vi "CounterCountEdgePulseSync.vi"() -> ()   [LabVIEW 2023]
uses:
  <vilib>/Utility/error.llb/DialogType.ctl
  <vilib>/DAQmx/read.llb/DAQmx Read (Counter 1D DBL 1Chan NSamp).vi
  <vilib>/DAQmx/create/channels.llb/DAQmx Create Channel (CI-Count Edges).vi
  <vilib>/DAQmx/create/channels.llb/DAQmx Create Channel (CO-Pulse Generation-Time).vi
  <vilib>/DAQmx/create/channels.llb/DAQmx Create Channel (AI-Voltage-Basic).vi
  <vilib>/DAQmx/configure/timing.llb/DAQmx Timing (Sample Clock).vi
  <vilib>/DAQmx/configure/timing.llb/DAQmx Timing (Implicit).vi
  <vilib>/DAQmx/miscellaneous.llb/DAQmx Fill In Error Info.vi
  <resource>/objmgr/daqmx.rc
panel:
  in  "# of pulses":i32=1000
  in  "Pulse Output terminal":tag
  in  "CI.CountEdges.Term":tag
  out "data":dbl[](array[numeric]) caption="Counter 0 Data" format="%0.2f"
  in  "Sample Clock Source":tag="/Dev1/ai/SampleClock"
  in  "rate":dbl=1000.0 format="%0.2f"
  in  "Physical Channel":tag="Dev1/ai0"
  in  "active edge":i32(ring)=10280 items=["Rising"=10280, "Falling"=10171]
  in  "Physical Channel":tag="Dev1/ctr1"
  in  "Physical Channel":tag="Dev1/ctr0"
  in  "stop":bool
  # "Analog Channel Properties"
  # "Counter 0 Channel Properties"
  # "Counter 1 Channel Properties"
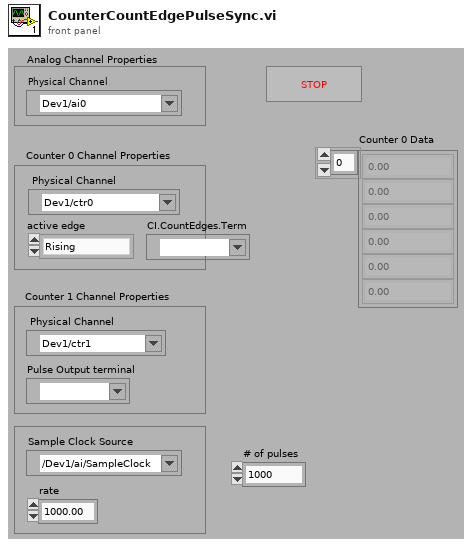
[diagram p1: front panel]
types:
  T1 = typedef "DialogType.ctl" = u16
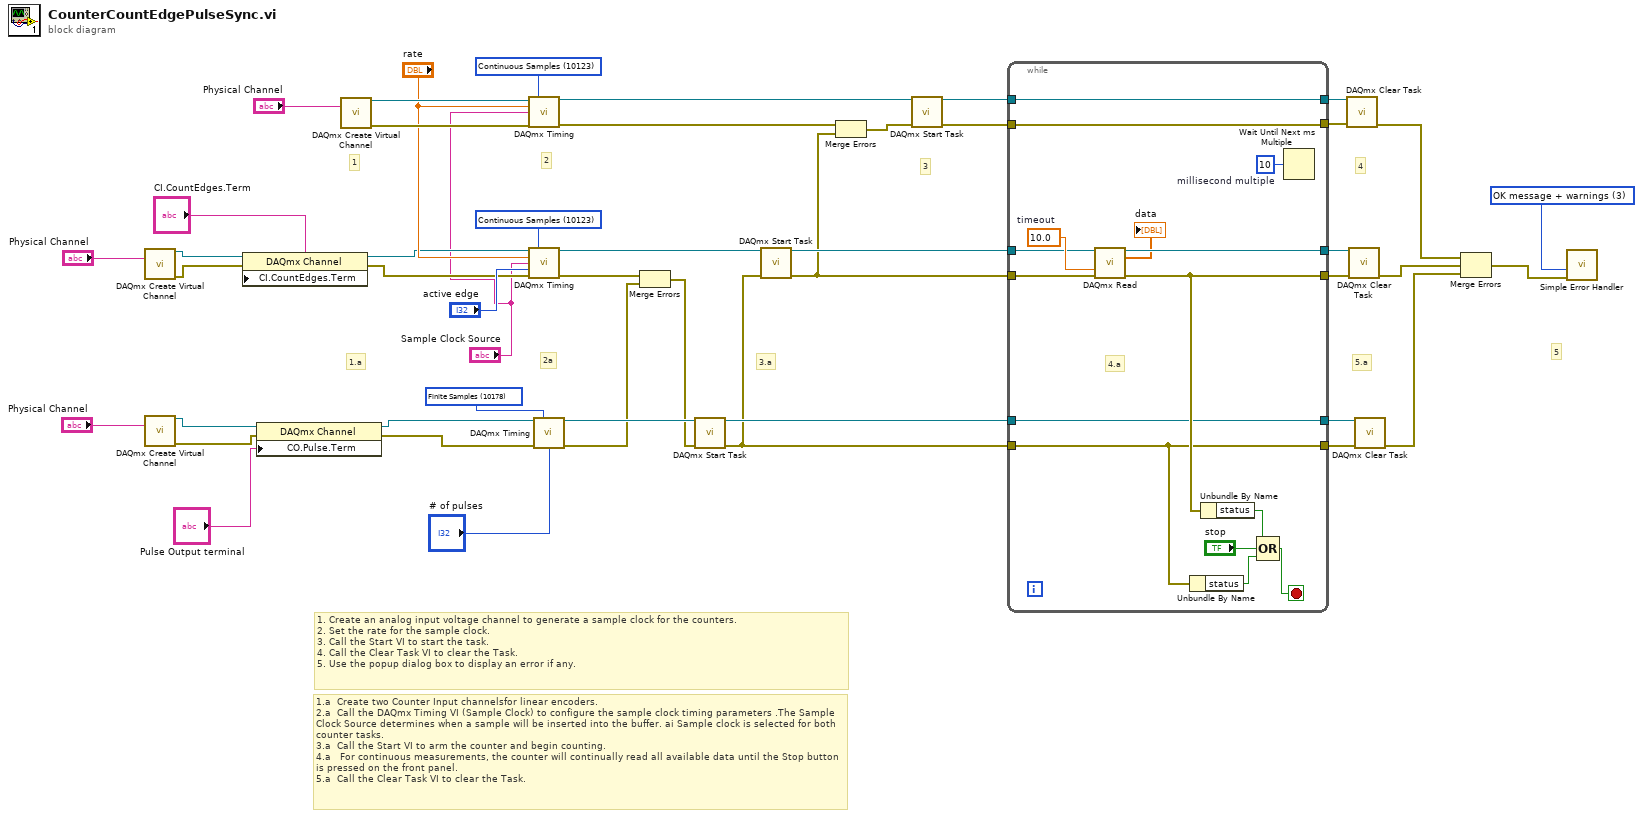
[diagram p0: block diagram]
diagram:
  w13 = 10123 items=["Finite Samples"=10178, "Continuous Samples"=10123, "Hardware Timed Single Point"=12522] ("sample mode")
  w14 = 10178 items=["Finite Samples"=10178, "Continuous Samples"=10123, "Hardware Timed Single Point"=12522] ("sample mode")
  w15 = 10123 items=["Finite Samples"=10178, "Continuous Samples"=10123, "Hardware Timed Single Point"=12522] ("sample mode")
  w33 = T1 3 items=["no dialog", "OK message", "continue or stop message", "OK message + warnings", "continue/stop + warnings"] ("type of dialog (OK msg:1)")
  # "1. Create an analog input voltage channel to generate a sample clock for the counters.\n2. Set the rate for the sample clock.\n3. Call the Start VI to start the task.\n4. Call the Clear Task VI to clear the Task.\n5. Use the popup dialog box to display an error if any."
  # "5"
  # "1.a  Create two Counter Input channelsfor linear encoders. \n2.a  Call the DAQmx Timing VI (Sample Clock) to configure the sample clock timing parameters .The Sample Clock Source determines when a sample will be inserted into the buffer. ai Sample clock is selected for both counter tasks.\n3.a  Call the Start VI to arm the counter and begin counting.\n4.a   For continuous measurements, the counter will continually read all available data until the Stop button is pressed on the front panel.\n5.a  Call the Clear Task VI to clear the Task."
  # "5.a"
  # "3.a"
  # "2a"
  # "1.a"
  # "4"
  # "3"
  # "2"
  # "1"
  n1 = call-poly <vilib>:"DAQmx Create Virtual Channel.vi"("counter"="Physical Channel") -> ("task out"=w12:refnum<k21>, "error out"=w9:errorcluster)  [unwired: 6 in, 7 out]
  n2 = call-poly <vilib>:"DAQmx Create Virtual Channel.vi"("counter"="Physical Channel") -> ("task out"=w7:refnum<k21>, "error out"=w4:errorcluster)  [unwired: 8 in, 5 out]
  n3 = property class="DAQmx Channel"(reference=w12, error in=w9, "CI.CountEdges.Term"="CI.CountEdges.Term") -> (reference out=w11:refnum<k21>, error out=w10:errorcluster)
  n4 = property class="DAQmx Channel"(reference=w7, error in=w4, "CO.Pulse.Term"="Pulse Output terminal") -> (reference out=w6:refnum<k21>, error out=w5:errorcluster)
  n5 = call-poly <vilib>:"DAQmx Create Virtual Channel.vi"("physical channels"="Physical Channel") -> ("task out"=w47:refnum<k21>, "error out"=w46:errorcluster)  [unwired: 8 in, 5 out]
  n6 = call-poly <vilib>:"DAQmx Timing.vi"("task/channels in"=w47, "sample mode"=w15, "rate"="rate", "source"="Sample Clock Source", "error in"=w46) -> ("task out"=w41:refnum<k21>, "error out"=w37:errorcluster)  [unwired: 2 in, 7 out]
  n7 = call-poly <vilib>:"DAQmx Timing.vi"("task/channels in"=w11, "sample mode"=w13, "rate"="rate", "source"="Sample Clock Source", "active edge"="active edge", "error in"=w10) -> ("task out"=w43:refnum<k21>, "error out"=w40:errorcluster)  [unwired: 1 in, 7 out]
  n8 = call-poly <vilib>:"DAQmx Timing.vi"("task/channels in"=w6, "sample mode"=w14, "samples per channel"="# of pulses", "error in"=w5) -> ("task out"=w42:refnum<k21>, "error out"=w38:errorcluster)  [unwired: 4 in, 6 out]
  n9 = Merge Errors(w40, w38) -> (w39:errorcluster)
  n10 = call <vilib>:"DAQmx Start Task.vi"("task/channels in"=w42, "error in"=w39) -> ("task out"=w28:refnum<k21>, "error out"=w27:errorcluster)  [unwired: 12 out]
  n11 = call <vilib>:"DAQmx Start Task.vi"("task/channels in"=w43, "error in"=w27) -> ("task out"=w30:refnum<k21>, "error out"=w29:errorcluster)  [unwired: 12 out]
  n12 = Merge Errors(w37, w29) -> (w36:errorcluster)
  n13 = call <vilib>:"DAQmx Start Task.vi"("task/channels in"=w41, "error in"=w36) -> ("task out"=w26:refnum<k21>, "error out"=w25:errorcluster)  [unwired: 12 out]
  n14 = while {
    tunnel: w29 -> [w62]
    tunnel: [w55] -> w35
    tunnel: [w58] -> w34
    tunnel: w28 -> [w54]
    tunnel: w27 -> [w53]
    tunnel: [w54] -> w32
    tunnel: [w53] -> w31
    tunnel: w30 -> [w52]
    tunnel: w26 -> [w51]
    tunnel: w25 -> [w50]
    tunnel: [w51] -> w24
    tunnel: [w50] -> w23
    stop <- w61 stop-if-true
    w56 = u32 10  # millisecond multiple
    w57 = 10.0  # timeout
    # "4.a"
    n15 = call-poly <vilib>:"DAQmx Read.vi"("task/channels in"=w52, "timeout"=w57, "error in"=w62) -> ("task out"=w58:refnum<k21>, "data"=→"data":dbl[], "error out"=w55:errorcluster)  [unwired: 1 in, 9 out]
    n16 = Unbundle By Name(w53) -> ("status"=w49:bool)
    n17 = Unbundle By Name(w55) -> ("status"=w59:bool)
    n18 = Compound Arithmetic op=OR(w59, "stop", w49) -> (w61:bool)
    n19 = Wait Until Next ms Multiple(millisecond multiple=w56) -> ()  [unwired: 1 out]
  }
  n20 = call <vilib>:"DAQmx Clear Task.vi"("task in"=w24, "error in"=w23) -> ("error out"=w21:errorcluster)  [unwired: 13 out]
  n21 = call <vilib>:"DAQmx Clear Task.vi"("task in"=w34, "error in"=w35) -> ("error out"=w22:errorcluster)  [unwired: 13 out]
  n22 = call <vilib>:"DAQmx Clear Task.vi"("task in"=w32, "error in"=w31) -> ("error out"=w20:errorcluster)  [unwired: 13 out]
  n23 = Merge Errors(w21, w22, w20) -> (w19:errorcluster)
  n24 = call <vilib>:"Simple Error Handler.vi"("type of dialog (OK msg:1)"=w33, "error in (no error)"=w19) -> ()  [unwired: 8 out]
